vi "OCR_Select Rectangle.vi"(8 "Error":errorcluster, 9 "Region":T2, 11 "2D Image":T1) -> (0 "Error Out":errorcluster, 3 "2D Image Out":T1)   [LabVIEW 2009]
doc: "Selects a portion of the 2D image"
uses:
  Controls/Array/Color Box Array_2D Icon Viewer.ctl
  Controls/Cluster/Cluster_Region info.ctl
  Controls/Cluster/Cluster_Top Left position.ctl
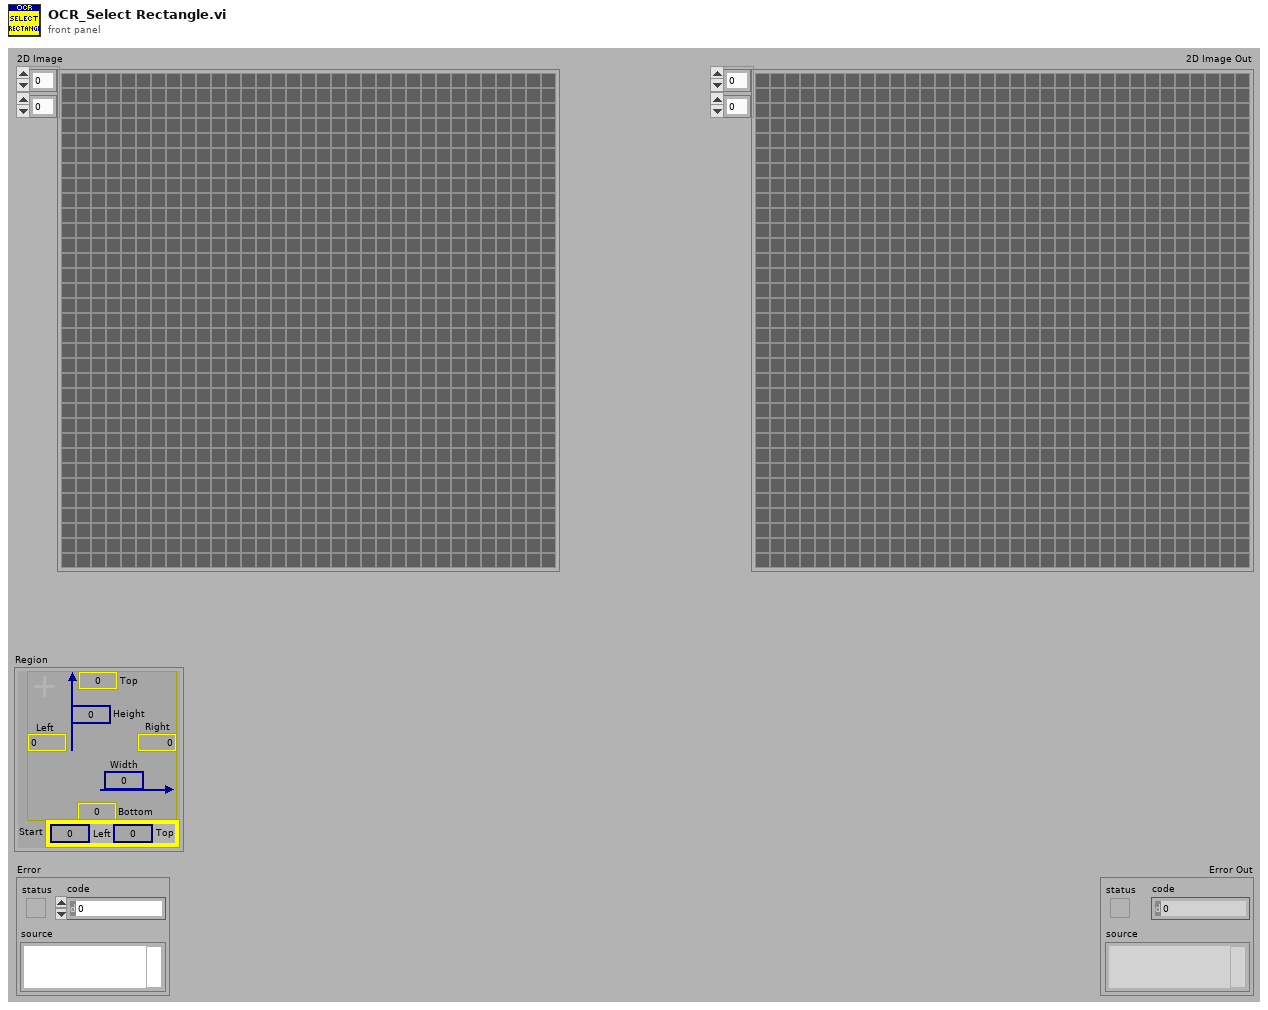
[diagram p1: front panel]
types:
  T1 = typedef "Color Box Array_2D Icon Viewer.ctl" = u32[][]
  T2 = typedef "Cluster_Region info.ctl" = cluster{"Left":i32, "Top":i32, "Right":i32, "Bottom":i32, "Width":u32, "Height":u32, "Start":T3}
  T3 = typedef "Cluster_Top Left position.ctl" = cluster{"Left":i32, "Top":i32}
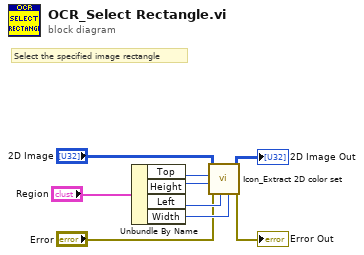
[diagram p0: block diagram]
diagram:
  # "Select the specified image rectangle"
  n1 = Unbundle By Name("Region") -> ("Top"=w9:i32, "Height"=w8:u32, "Left"=w7:i32, "Width"=w6:u32)
  n2 = call "Icon_Extract 2D color set.vi"("Width"=w6, "Left"=w7, "Error"="Error", "Height"=w8, "Top"=w9, "2D Image"="2D Image") -> ("Error Out"=→"Error Out":errorcluster, "2D Image Out"=→"2D Image Out":T1)  [unwired: 4 in]
